vi "FTW-Connector-Tell.vi"(0 "FTW Actor Connector":refnum<class "FTW-ActorConnector.lvclass">, 5 "Message Header":string, 7 "Message Body":string, 9 "Timeout":i32 format="%dmsec", 11 "error in":errorcluster) -> (4 "FTW Actor Connector out":refnum<class "FTW-ActorConnector.lvclass">, 6 "Timed out?":bool, 15 "error out":errorcluster)   [LabVIEW 2012, in "FTW-Actor.lvlib" / "FTW-ActorConnector.lvclass"]
uses:
  FTW-ActorConnector.lvclass
  FTW-ActorConnector.lvclass/FTW-ActorConnector.ctl
  Endpoint/FTW-Endpoint.lvclass
panel:
  # "Inputs"
  # "Outputs"
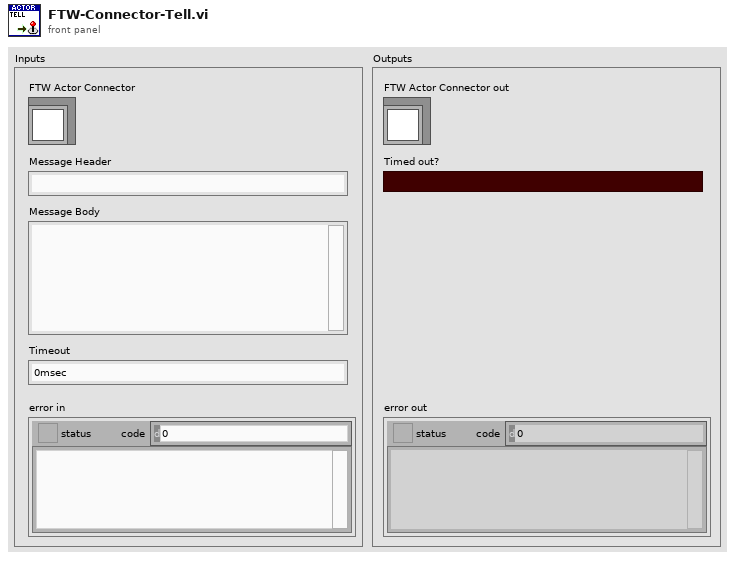
[diagram p1: front panel]
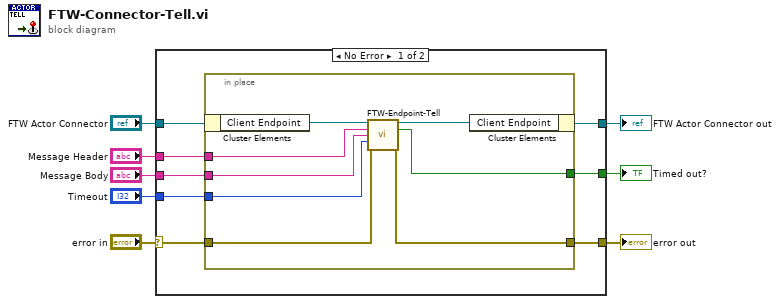
[diagram p0: block diagram]
diagram:
  n1 = case shown="No Error" "error in" {
    selector: "error in" -> [w15 w26]
    tunnel: [w13 w26] -> w7
    tunnel: "FTW Actor Connector" -> [w16 w25]
    tunnel: [w14 w25] -> w5
    tunnel: "Message Header" -> [w12 _]
    tunnel: "Message Body" -> [w11 _]
    tunnel: "Timeout" -> [w10 _]
    tunnel: [w9 _] -> w1
    frame No Error {
      n2 = in-place {
        in-place-border: w15 -> [w24]
        in-place-border: [w23] -> w13
        in-place-border: w12 -> [w20]
        in-place-border: w11 -> [w19]
        in-place-border: w10 -> [w18]
        in-place-border: [w17] -> w9
        n3 = in-place-cluster #1(w16) -> ("Client Endpoint"=w22:refnum<class "FTW-Endpoint.lvclass">)
        n4 = call-dynamic "FTW-Endpoint-Tell.vi"("FTW Endpoint"=w22, "Message Header"=w20, "Message Body"=w19, "Timeout"=w18, "error in"=w24) -> ("FTW Endpoint out"=w21:refnum<class "FTW-Endpoint.lvclass">, "Timed out?"=w17:bool, "error out"=w23:errorcluster)  [unwired: 8 in]
        n5 = in-place-cluster #1("Client Endpoint"=w21) -> (w14:refnum<class "FTW-ActorConnector.lvclass">)
      }
    }
    frame Error {
    }
  }
  "error out" <- w7
  "FTW Actor Connector out" <- w5
  "Timed out?" <- w1
